vi "Mask to Alpha.vi"(11 "image data":T1) -> (3 "image data out":T1)   [LabVIEW 2021, in "TSC Material Theme.lvlib" / "Material-Scheme.lvclass"]
doc: "convert mask data to alpha layer\n\n<b>Code Developed By:</b>\nTechnology Service Corporation\nwww.tsc.com/atcs\n\nDeveloper:\nDaniel Coons"
uses:
  Material-Scheme.lvclass
  <vilib>/picture/picture.llb/imagedata.ctl
  Material-Scheme.lvclass/Material-Scheme.ctl
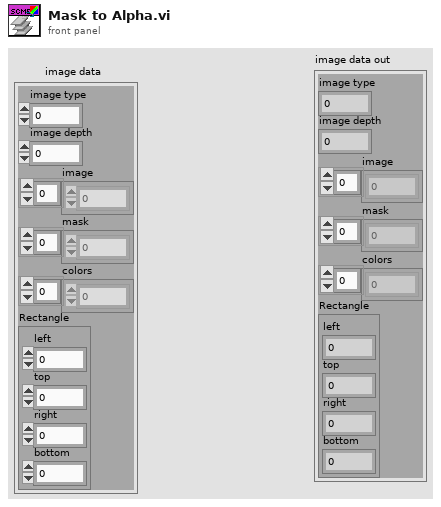
[diagram p1: front panel]
types:
  T1 = typedef "imagedata.ctl" = cluster{"image type":i32, "image depth":i32, "image":u8[], "mask":u8[], "colors":u32[], "Rectangle":cluster{"left":i16, "top":i16, "right":i16, "bottom":i16}}
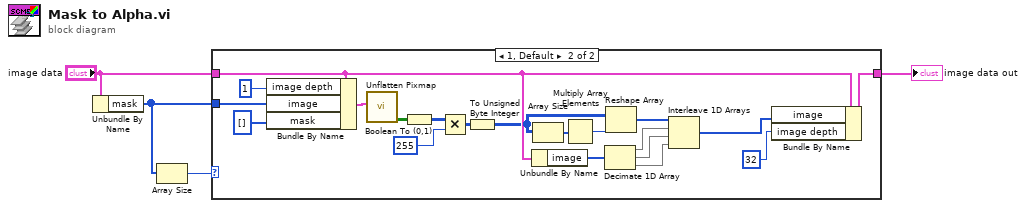
[diagram p0: block diagram]
diagram:
  n1 = Unbundle By Name("image data") -> ("mask"=w3:u8[])
  n2 = Array Size(array=w3) -> (size(s)=w2:i32)
  n3 = case shown="1, Default" w2 {
    tunnel: "image data" -> [w5 w15]
    tunnel: w3 -> [_ w18]
    tunnel: [w5 w14] -> w1
    frame 0 {
    }
    frame 1, Default {
      n4 = Bundle By Name(cluster=w15, "image depth"=1, "image"=w18, "mask"=u8[] []) -> (w25:T1)
      n5 = call <vilib>:"Unflatten Pixmap.vi"("image data"=w25) -> ("1-bit pixmap"=w22:bool[][])  [unwired: 4 in, 6 out]
      n6 = Boolean To (0,1)(Boolean=w22) -> (0, 1=w21:i16[][])
      n7 = Multiply(x=w21, y=255) -> (x*y=w19:i32[][])
      n8 = To Unsigned Byte Integer(number=w19) -> (unsigned 8bit integer=w11:u8[][])
      n9 = Unbundle By Name(w15) -> ("image"=w12:u8[])
      n10 = Array Size(array=w11) -> (size(s)=w17:i32[])
      n11 = Multiply Array Elements(1:w17) -> (0:w16:i32)
      n12 = Decimate 1D Array(w12) -> (w9:u8[], w8:u8[], w7:u8[])
      n13 = Reshape Array(w11, w16) -> (w10:u8[])
      n14 = Interleave 1D Arrays(w10, w9, w8, w7) -> (w6:u8[])
      n15 = Bundle By Name(cluster=w15, "image"=w6, "image depth"=32) -> (w14:T1)
    }
  }
  "image data out" <- w1
